vi "Wait for VeriStand Host.vi"   [LabVIEW 2019]
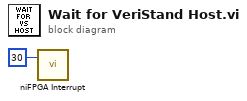
[diagram p0: block diagram]
diagram:
  n1 = call <vilib>:"niFPGA Interrupt.vi"("IRQ Number (0)"=u8 30) -> ()  [unwired: 2 in]
